vi "ENTROdll.vi"(8 "error in (no error)":errorcluster, 9 "z":dbl[](array[numeric]), 10 "D":dbl, 11 "t":dbl) -> (0 "error out":errorcluster, 3 "s":dbl)   [LabVIEW 2016]
doc: "subroutine ENTROdll(t, D, z, s)\n\nCompute entropy as a function of temperature, density and composition\nusing core functions (temperature derivative of Helmholtz free energy\nand ideal gas integrals)\n\nbased on derivations in Younglove & McLinden, JPCRD 23 #5, 1994,\nequations A5, A19 - A26\n\nINPUTS:\nt -- temperature [K]\nD -- molar density [mol/L]\nz -- composition [array of mol frac]\n\nOUTPUTS:\ns -- entropy [J/mol-K]"
uses:
  REFPROP.DLL
panel:
  # "REFPROP-ENTROdll.vi"
  # "void  ENTROdll(double *t, double *D, double *z, double *s)"
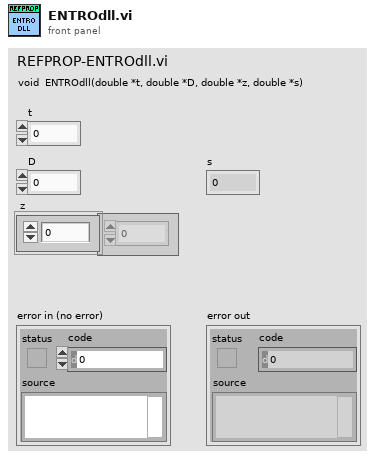
[diagram p1: front panel]
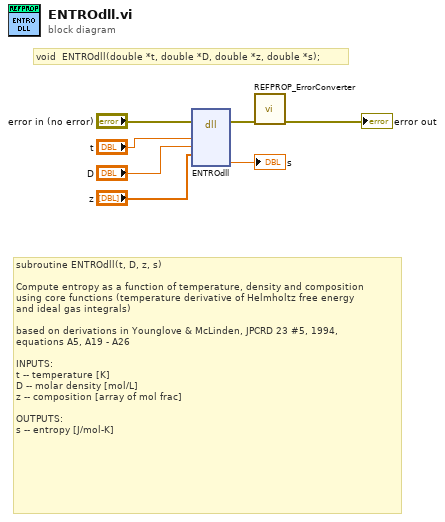
[diagram p0: block diagram]
diagram:
  # "void  ENTROdll(double *t, double *D, double *z, double *s);"
  # "subroutine ENTROdll(t, D, z, s)\n\nCompute entropy as a function of temperature, density and composition\nusing core functions (temperature derivative of Helmholtz free energy\nand ideal gas integrals)\n\nbased on derivations in Younglove & McLinden, JPCRD 23 #5, 1994,\nequations A5, A19 - A26\n\nINPUTS:\nt -- temperature [K]\nD -- molar density [mol/L]\nz -- composition [array of mol frac]\n\nOUTPUTS:\ns -- entropy [J/mol-K]"
  n1 = dll-call lib="S:/009 - Testing/02 - Performance Testing/REFPROP/REFPROP.*" fn="ENTROdll"(error in="error in (no error)", "t"="t", "D"="D", "z"="z") -> (error out=w3:errorcluster, "s"=→"s":dbl)  [unwired: 7 in, 1 out]
  n2 = call "REFPROP_ErrorConverter.vi"("error in (no error)"=w3) -> ("error out"=→"error out":errorcluster)  [unwired: 10 in]
